vi "3_adder.vi"(4 "y":dbl, 6 "x":dbl, 7 "x 3":dbl, 9 "y 2":dbl, 10 "x 2":dbl, 11 "y 3":dbl) -> (1 "Numeric":dbl, 2 "Numeric 2":dbl, 3 "Numeric 3":dbl)   [LabVIEW 2021]
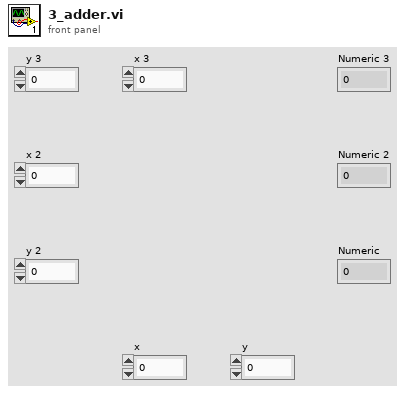
[diagram p1: front panel]
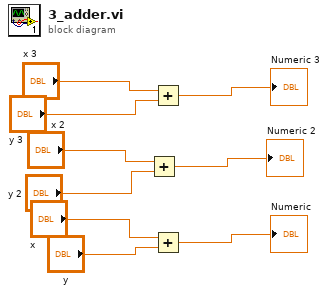
[diagram p0: block diagram]
diagram:
  n1 = Add(x="x 2", y="y 2") -> (x+y=→"Numeric 2":dbl)
  n2 = Add(x="x 3", y="y 3") -> (x+y=→"Numeric 3":dbl)
  n3 = Add(x="x", y="y") -> (x+y=→"Numeric":dbl)
